vi "Get Waveform.vi"(8 "error in (no error)":errorcluster, 10 "Save data":bool, 11 "Tektronix MSO 6 Driver in":refnum<class "Tektronix MSO 6 Driver.lvclass">) -> (0 "error out":errorcluster, 2 "Waveform":waveform(dbl), 3 "Tektronix MSO 6 Driver out":refnum<class "Tektronix MSO 6 Driver.lvclass">)   [LabVIEW 2020, in "Tektronix MSO 6 Driver.lvclass"]
uses:
  Tektronix MSO 6 Driver.lvclass
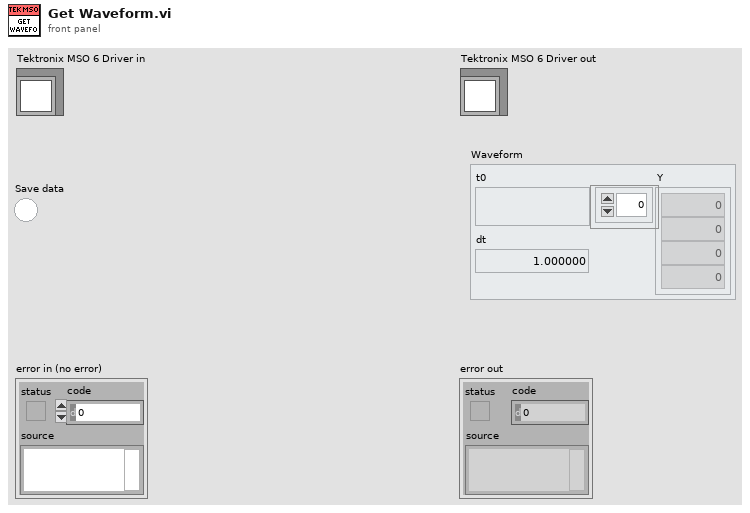
[diagram p1: front panel]
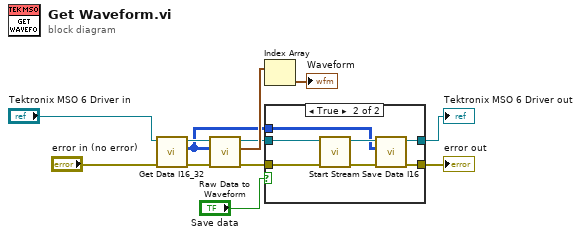
[diagram p0: block diagram]
diagram:
  n1 = call-dynamic "Get Data I16_32.vi"("error in (no error)"="error in (no error)", "Tektronix MSO 6 Driver in"="Tektronix MSO 6 Driver in") -> ("error out"=w11:errorcluster, "I16 data out"=w3:i16[][], "Tektronix MSO 6 Driver out"=w12:refnum<class "Tektronix MSO 6 Driver.lvclass">)  [unwired: 4 in, 3 out]
  n2 = call-dynamic "Raw Data to Waveform.vi"("error in (no error)"=w11, "I16 data"=w3, "Pulse Driver in"=w12) -> ("error out"=w4:errorcluster, "Array"=w8:waveform(dbl)[], "Pulse Driver out"=w5:refnum<class "Tektronix MSO 6 Driver.lvclass">)  [unwired: 6 in]
  n3 = Index Array(array=w8) -> (element=→"Waveform":waveform(dbl))  [unwired: 1 in]
  n4 = case shown="True" "Save data" {
    tunnel: w5 -> [w14 w21]
    tunnel: w4 -> [w13 w20]
    tunnel: w3 -> [_ w17]
    tunnel: [w14 w16] -> w2
    tunnel: [w13 w15] -> w1
    frame False {
    }
    frame True {
      n5 = call-dynamic "Start Stream.vi"("error in (no error)"=w20, "Pulse Driver in"=w21) -> ("error out"=w18:errorcluster, "Pulse Driver out"=w19:refnum<class "Tektronix MSO 6 Driver.lvclass">)  [unwired: 8 in]
      n6 = call-dynamic "Save Data I16.vi"("error in (no error)"=w18, "I16 data"=w17, "Pulse Driver in"=w19) -> ("error out"=w15:errorcluster, "Pulse Driver out"=w16:refnum<class "Tektronix MSO 6 Driver.lvclass">)  [unwired: 7 in]
    }
  }
  "error out" <- w1
  "Tektronix MSO 6 Driver out" <- w2
